vi "Comparison.vi"() -> ()   [LabVIEW 2014]
panel:
  out "Win second":u8(slide) scale=0.0..100.0
  out "Win first":u8(slide) scale=0.0..100.0
  in  "Next comparison":bool
  out "Second number":dbl
  out "First number":dbl
  out "Fn>Sn":bool
  in  "stop":bool
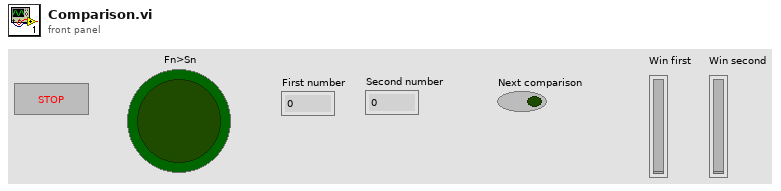
[diagram p1: front panel]
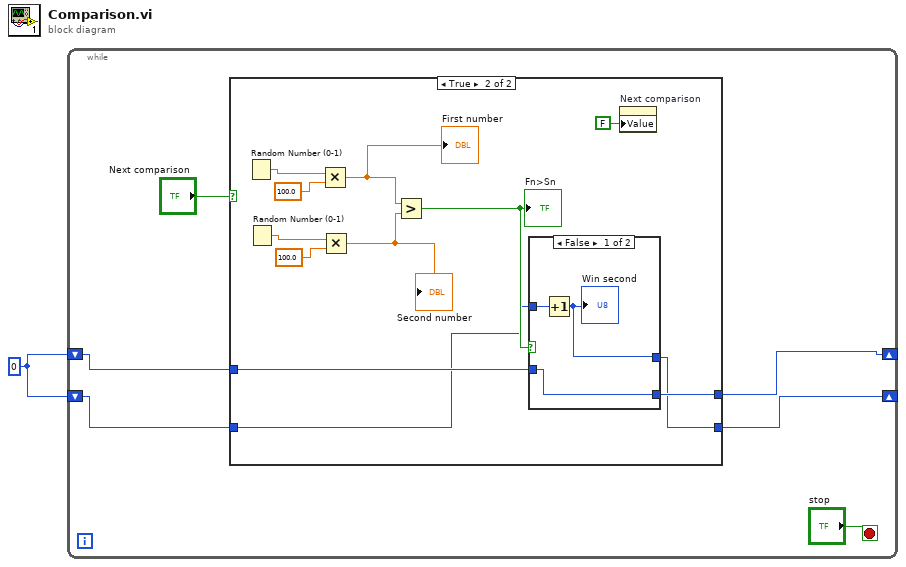
[diagram p0: block diagram]
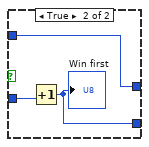
[diagram p3: hidden frame]
diagram:
  w1 = 0
  n1 = while {
    shift-right: [w4] -> _
    shift-left: w1 -> [w5]
    shift-right: [w2] -> _
    shift-left: w1 -> [w3]
    stop <- "stop" stop-if-true
    n2 = case shown="True" "Next comparison" {
      tunnel: w5 -> [w9 w13]
      tunnel: [w9 w12] -> w4
      tunnel: w3 -> [w8 w11]
      tunnel: [w8 w10] -> w2
      frame False {
      }
      frame True {
        n3 = Random Number (0-1)() -> (number: 0 to 1=w21:dbl)
        n4 = Random Number (0-1)() -> (number: 0 to 1=w18:dbl)
        n5 = Multiply(x=w21, y=100.0) -> (x*y=w16:dbl)
        "First number" <- w16
        n6 = Multiply(x=w18, y=100.0) -> (x*y=w17:dbl)
        "Second number" <- w17
        n7 = Greater?(x=w16, y=w17) -> (0:w14:bool)
        "Fn>Sn" <- w14
        n8 = case shown="False" w14 {
          tunnel: w13 -> [w24 w27]
          tunnel: [w24 w26] -> w12
          tunnel: w11 -> [w23 w25]
          tunnel: [w22 w25] -> w10
          frame False {
            n9 = Increment(x=w23) -> (x+1=w22:i32)
            "Win second" <- w22
          }
          frame True {
            n10 = Increment(x=w27) -> (x+1=w26:i32)
            "Win first" <- w26
          }
        }
        n11 = property on="Next comparison" class="Bool (strict)"("Value"=FALSE ("Next comparison")) -> ()  [unwired: 2 in, 2 out]
      }
    }
  }
